vi "User Management (Subvi).vi"() -> ()   [LabVIEW 2009]
uses:
  <vilib>/Utility/file.llb/Read From Spreadsheet File (string).vi
  <vilib>/Utility/file.llb/Write To Spreadsheet File (string).vi
panel:
  in  "Change":bool
  in  "Delete":bool
  in  "Multicolumn Listbox":i32(listbox)
  in  "Type":string(combo)="Student"
  in  "stop":bool
  in  "Create":bool
  in  "Password":string
  in  "Username":string
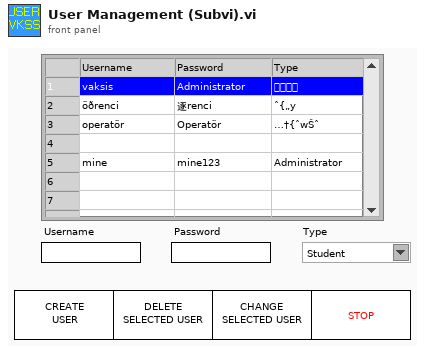
[diagram p1: front panel]
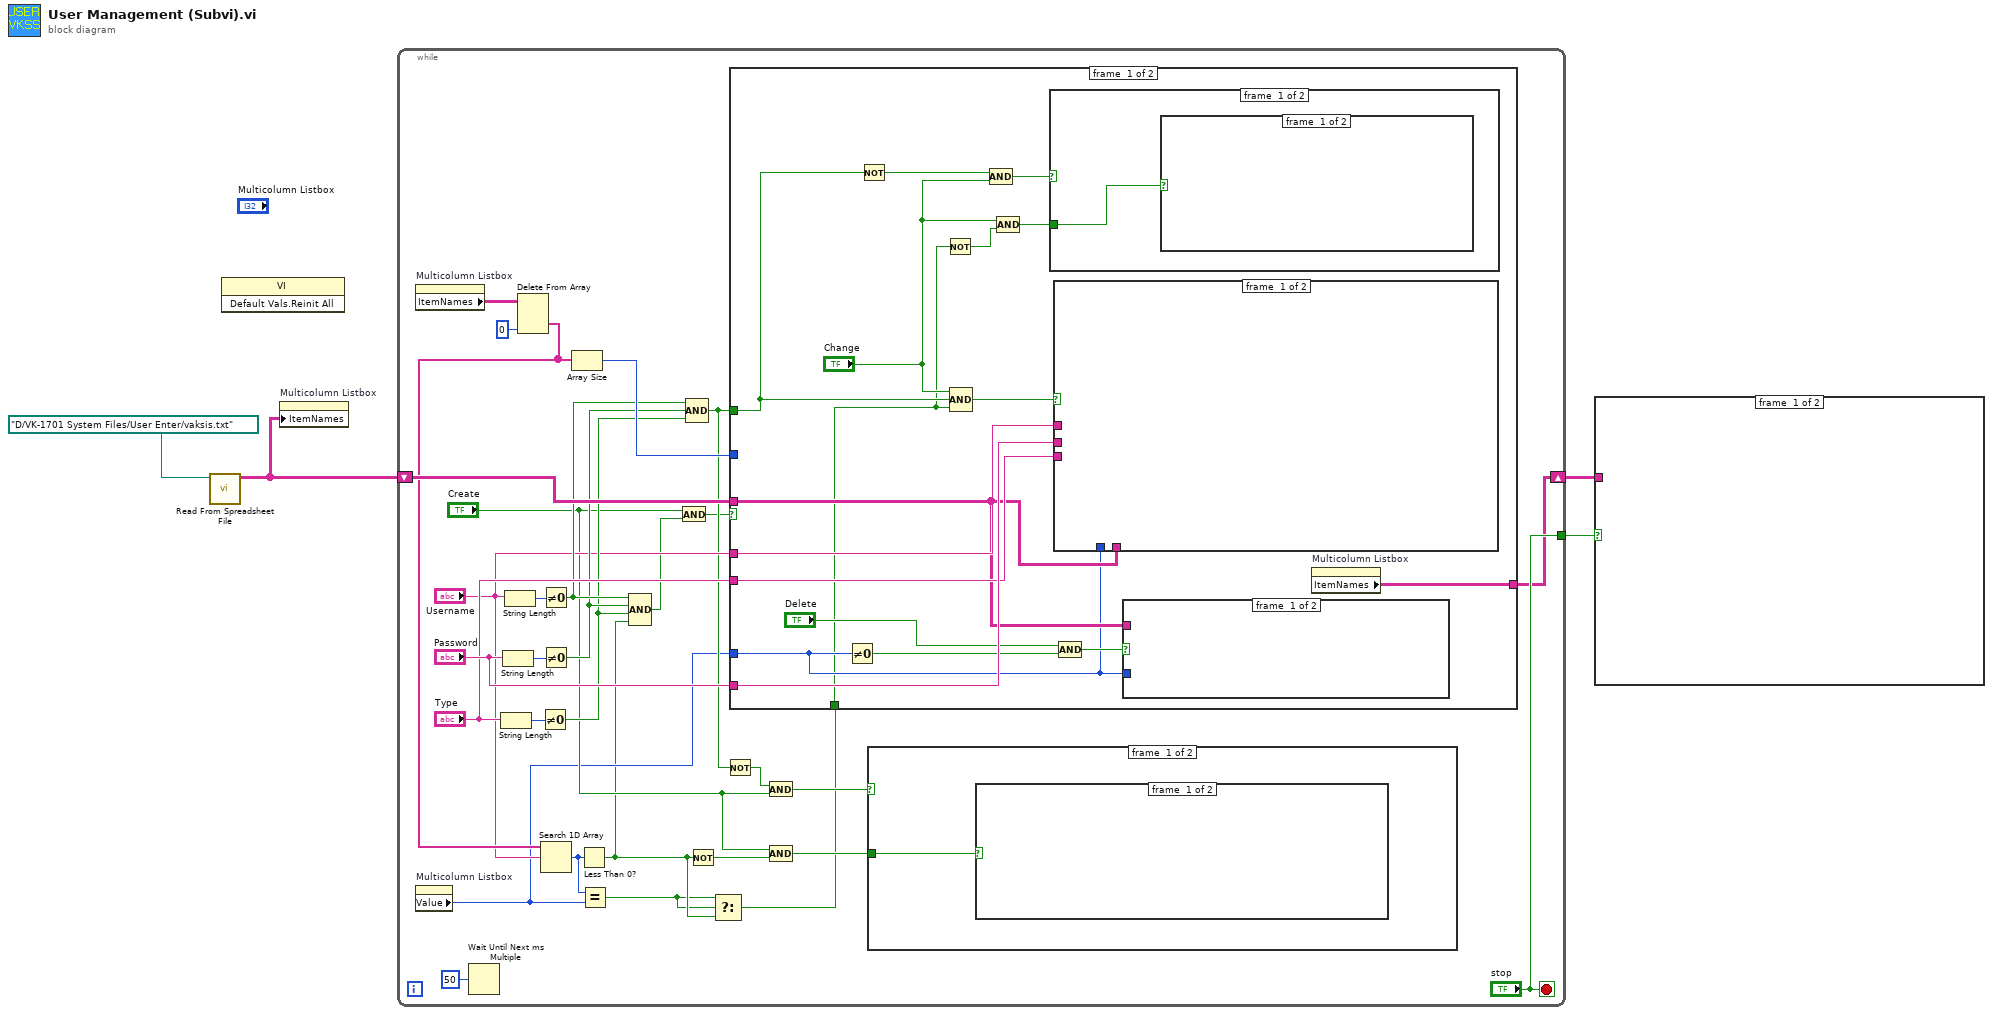
[diagram p0: block diagram]
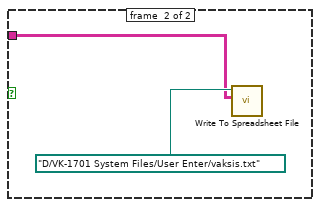
[diagram p2: hidden frame]
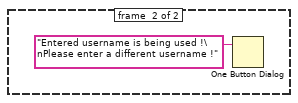
[diagram p3: hidden frame]
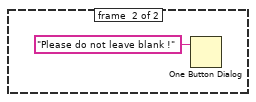
[diagram p4: hidden frame]
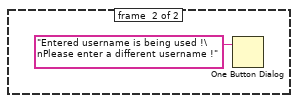
[diagram p5: hidden frame]
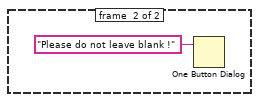
[diagram p6: hidden frame]
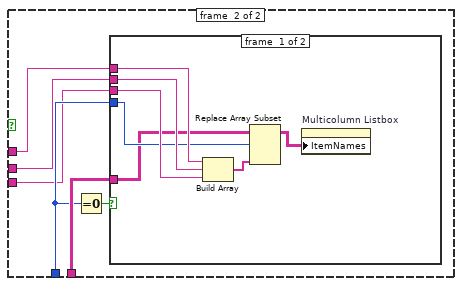
[diagram p7: hidden frame]
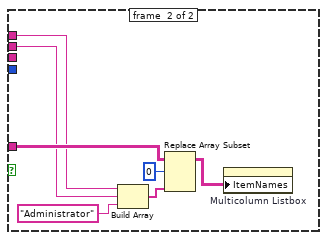
[diagram p8: hidden frame]
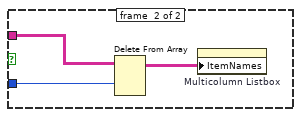
[diagram p9: hidden frame]
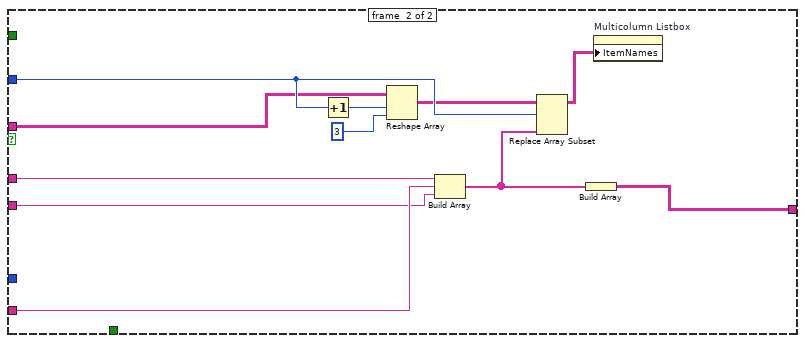
[diagram p10: hidden frame]
diagram:
  n1 = call-poly <vilib>:"Read From Spreadsheet File.vi"("file path (dialog if empty)"=path "D:/VK-1701 System Files/User Enter/vaksis.txt" ("file (use dialog) 2")) -> ("all rows"=w1:string[][])  [unwired: 6 in, 4 out]
  n2 = invoke class="VI" method="Default Vals.Reinit All"() -> ()  [unwired: 3 in, 3 out]
  n3 = property on="Multicolumn Listbox" class="MCListbox (strict)"("ItemNames"=w1) -> ()  [unwired: 2 in, 2 out]
  n4 = while {
    shift-right: [w30] -> w3
    shift-left: w1 -> [w32]
    tunnel: ["stop"] -> w2
    stop <- "stop" stop-if-true
    n5 = property on="Multicolumn Listbox" class="MCListbox (strict)"() -> ("ItemNames"=w23:string[][])  [unwired: 2 in, 2 out]
    n6 = property on="Multicolumn Listbox" class="MCListbox (strict)"() -> ("Value"=w8:i32)  [unwired: 2 in, 2 out]
    n7 = Wait Until Next ms Multiple(millisecond multiple=u32 50) -> ()  [unwired: 1 out]
    n8 = String Length(string="Type") -> (length=w28:i32)
    n9 = String Length(string="Password") -> (length=w27:i32)
    n10 = String Length(string="Username") -> (length=w29:i32)
    n11 = Delete From Array(array=w23, index (col)=0 ("disabled index (col)")) -> (deleted portion=w18:string[])  [unwired: 2 in, 1 out]
    n12 = Not Equal To 0?(x=w28) -> (x != 0?=w19:bool)
    n13 = Not Equal To 0?(x=w29) -> (x != 0?=w21:bool)
    n14 = Not Equal To 0?(x=w27) -> (x != 0?=w20:bool)
    n15 = Search 1D Array(1D array=w18, element="Username") -> (index of element=w9:i32)  [unwired: 1 in]
    n16 = Array Size(array=w18) -> (size(s)=w22:i32)
    n17 = Less Than 0?(x=w9) -> (x < 0?=w7:bool)
    n18 = Equal?(x=w9, y=w8) -> (x = y?=w6:bool)
    n19 = Compound Arithmetic op=AND(w21, w20, w19, w7) -> (w11:bool)
    n20 = And(x="Create", y=w11) -> (x .and. y?=w12:bool)
    n21 = Compound Arithmetic op=AND(w21, w20, w19) -> (w16:bool)
    n22 = Not(x=w7) -> (.not. x?=w15:bool)
    n23 = Select(t=w6, s=w6, f=w7) -> (s? t:f=w5:bool)
    n24 = Not(x=w16) -> (.not. x?=w24:bool)
    n25 = case shown="False" w12 {
      tunnel: w22 -> [_ w85]
      tunnel: [w52 w86] -> w30
      tunnel: w32 -> [w50 w82]
      tunnel: "Username" -> [w54 w91]
      tunnel: "Password" -> [w53 w90]
      tunnel: "Type" -> [w51 w89]
      tunnel: w16 -> [w40 _]
      tunnel: w8 -> [w41 _]
      tunnel: w5 -> [w39 _]
      frame #0 {
        n26 = Not Equal To 0?(x=w41) -> (x != 0?=w47:bool)
        n27 = Not(x=w40) -> (.not. x?=w45:bool)
        n28 = Not(x=w39) -> (.not. x?=w38:bool)
        n29 = Compound Arithmetic op=AND("Change", w40, w39) -> (w49:bool)
        n30 = Compound Arithmetic op=AND(w45, "Change") -> (w44:bool)
        n31 = Compound Arithmetic op=AND("Change", w38) -> (w42:bool)
        n32 = case shown="False" w44 {
          tunnel: w42 -> [w55 _]
          frame #0 {
            n33 = case shown="True" w55 {
              frame #0 {
              }
              frame #1 {
                n34 = One Button Dialog(message="Entered username is being used !\nPlease enter a different username !") -> ()  [unwired: 1 in, 1 out]
              }
            }
          }
          frame #1 {
            n35 = One Button Dialog(message="Please do not leave blank !") -> ()  [unwired: 1 in, 1 out]
          }
        }
        n36 = case shown="True" w49 {
          tunnel: w50 -> [_ w62]
          tunnel: w54 -> [_ w61]
          tunnel: w53 -> [_ w60]
          tunnel: w41 -> [_ w59]
          tunnel: w51 -> [_ w58]
          frame #0 {
          }
          frame #1 {
            n37 = Equal To 0?(x=w59) -> (x = 0?=w63:bool)
            n38 = case shown="False" w63 {
              tunnel: w61 -> [w68 w73]
              tunnel: w60 -> [w67 w72]
              tunnel: w62 -> [w64 w77]
              tunnel: w59 -> [w65 _]
              tunnel: w58 -> [w66 _]
              frame #0 {
                n39 = Build Array(w68, w67, w66) -> (w70:string[])
                n40 = Replace Array Subset(array=w64, new element=w70, index (row)=w65) -> (w69:string[][])  [unwired: 1 in]
                n41 = property on="Multicolumn Listbox" class="MCListbox (strict)"("ItemNames"=w69) -> ()  [unwired: 2 in, 2 out]
              }
              frame #1 {
                n42 = Build Array(w73, w72, "Administrator" ("element")) -> (w76:string[])
                n43 = Replace Array Subset(array=w77, new element=w76, index (row)=0) -> (w74:string[][])  [unwired: 1 in]
                n44 = property on="Multicolumn Listbox" class="MCListbox (strict)"("ItemNames"=w74) -> ()  [unwired: 2 in, 2 out]
              }
            }
          }
        }
        n45 = Compound Arithmetic op=AND("Delete", w47) -> (w48:bool)
        n46 = case shown="True" w48 {
          tunnel: w50 -> [_ w78]
          tunnel: w41 -> [_ w79]
          frame #0 {
          }
          frame #1 {
            n47 = Delete From Array(array=w78, index (row)=w79) -> (array with subset deleted=w80:string[][])  [unwired: 2 in, 1 out]
            n48 = property on="Multicolumn Listbox" class="MCListbox (strict)"("ItemNames"=w80) -> ()  [unwired: 2 in, 2 out]
          }
        }
        n49 = property on="Multicolumn Listbox" class="MCListbox (strict)"() -> ("ItemNames"=w52:string[][])  [unwired: 2 in, 2 out]
      }
      frame #1 {
        n50 = Increment(x=w85) -> (x+1=w88:i32)
        n51 = Reshape Array(w82, w88, 3 ("dimension size")) -> (w81:string[][])
        n52 = Build Array(w91, w90, w89) -> (w87:string[])
        n53 = Replace Array Subset(array=w81, new element=w87, index (row)=w85) -> (w83:string[][])  [unwired: 1 in]
        n54 = Build Array(w87) -> (w86:string[][])
        n55 = property on="Multicolumn Listbox" class="MCListbox (strict)"("ItemNames"=w83) -> ()  [unwired: 2 in, 2 out]
      }
    }
    n56 = And(x=w24, y="Create") -> (x .and. y?=w14:bool)
    n57 = Compound Arithmetic op=AND("Create", w15) -> (w13:bool)
    n58 = case shown="False" w14 {
      tunnel: w13 -> [w35 _]
      frame #0 {
        n59 = case shown="True" w35 {
          frame #0 {
          }
          frame #1 {
            n60 = One Button Dialog(message="Entered username is being used !\nPlease enter a different username !") -> ()  [unwired: 1 in, 1 out]
          }
        }
      }
      frame #1 {
        n61 = One Button Dialog(message="Please do not leave blank !") -> ()  [unwired: 1 in, 1 out]
      }
    }
  }
  n62 = case shown="True" w2 {
    tunnel: w3 -> [_ w92]
    frame #0 {
    }
    frame #1 {
      n63 = call-poly <vilib>:"Write To Spreadsheet File.vi"("2D data"=w92, "file path (dialog if empty)"=path "D:/VK-1701 System Files/User Enter/vaksis.txt" ("file (use dialog)")) -> ()  [unwired: 6 in, 1 out]
    }
  }
